vi "applicaiton-globals.vi"() -> ()   [LabVIEW 2014]
panel:
  out "Running Flag":bool
  in  "Stop Application":bool
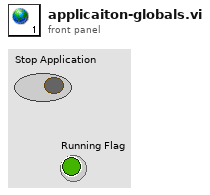
[diagram p1: front panel]
diagram:
